vi "Delete Controls.vi"(0 "Control in":refnum<vi>, 11 "error in (no error)":errorcluster) -> (15 "error out":errorcluster)   [LabVIEW 2021, in "Converter.lvlib"]
uses:
  Converter.lvlib
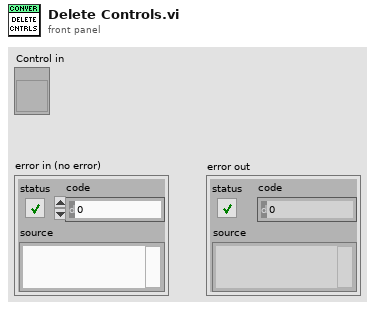
[diagram p1: front panel]
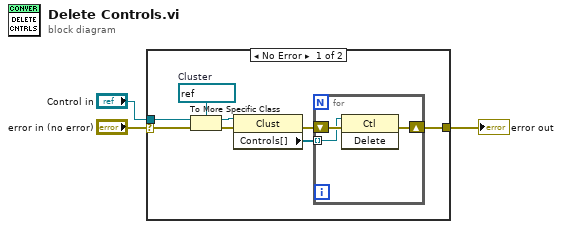
[diagram p0: block diagram]
diagram:
  n1 = case shown="No Error" "error in (no error)" {
    selector: "error in (no error)" -> [w4 w15]
    tunnel: [w11 w15] -> w3
    tunnel: "Control in" -> [w5 _]
    frame No Error {
      w6 = refnum<vi> refnum  # Cluster
      n2 = To More Specific Class(target class=w6, reference=w5, error in=w4) -> (specific class reference=w7:refnum<vi>, error out=w8:errorcluster)
      n3 = property class="Clust"(reference=w7, error in=w8) -> (error out=w9:errorcluster, "Controls[]"=w10:refnum<vi>[])  [unwired: 1 out]
      n4 = for {
        tunnel: w10 -> [w13] mode=indexing
        shift-right: [w12] -> w11
        shift-left: w9 -> [w14]
        n5 = invoke class="Ctl" method="Delete"(reference=w13, error in=w14) -> (error out=w12:errorcluster)  [unwired: 1 in, 2 out]
      }
    }
    frame Error {
    }
  }
  "error out" <- w3
